vi "Zan_OutBit.vi"(8 "error in (no error)":errorcluster, 10 "BL":bool, 11 "Zan IO_Output":T1) -> (0 "error out":errorcluster)   [LabVIEW 2015]
uses:
  Ctrl/Zan-64_SelectOutPut.ctl
  Ctrl/IO Card_Type.ctl
  global/IO_ClassTypeData.vi
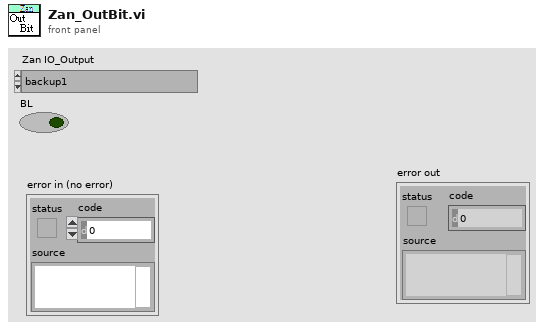
[diagram p1: front panel]
types:
  T1 = typedef "Zan-64_SelectOutPut.ctl" = enum16{"backup1", "ÎÌøQÆ÷", "¾¯Ê¾Ÿô(¾G)", "¾¯Ê¾Ÿô(üS)", "¾¯Ê¾Ÿô(¼t)", "ÉÏÒ•ÓX¹âÔ´", "ÏÂÒ•ÓX¹âÔ´", "ROBOTReadyӍ̖", "DUTQ±PÓÌ", "PASSQ±PÓÌ", "NGQ±PÓÌ", "ÒÆÝdÝSËÅ·þñRß_¼¤´Å"}
  T2 = typedef "IO Card_Type.ctl" = enum16{"None", "Unidaq32", "IPC_3005(9700)", "6480", "2410C-64", "Zan"}
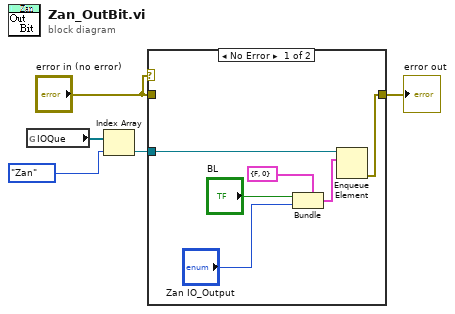
[diagram p0: block diagram]
diagram:
  n1 = global read "IO_ClassTypeData.vi" "IOQue"() -> (w3:refnum<queue>[])
  n2 = Index Array(array=w3, index=IO_Card_Type."Zan" ("IO Card Type")) -> (element=w1:refnum<queue>)
  n3 = case shown="No Error" "error in (no error)" {
    tunnel: "error in (no error)" -> [_ w12]
    tunnel: [w6 w12] -> w5
    tunnel: w1 -> [w11 _]
    frame No Error {
      n4 = Bundle(cluster=cluster{"BL":bool, "Index":i32} {"BL"=FALSE, "Index"=0} ("element"), "BL"="BL", "Index"="Zan IO_Output") -> (w8:cluster{"BL":bool, "Index":i32})
      n5 = Enqueue Element(queue=w11, element=w8) -> (error out=w6:errorcluster)  [unwired: 2 in, 2 out]
    }
    frame Error {
    }
  }
  "error out" <- w5
